vi "20220815-335-write temppoint.vi"() -> ()   [LabVIEW 2019]
doc: "This example VI demonstrates the proper use of the Configure Curve Header and Configure Curve Point VIs. It allows the user to write a curve header, a curve point, of both."
panel:
  out "当前已经写入（点数）":i32
  in  "曲线序号":string="59"
  in  "VISA resource name":refnum<visa-resource-name>
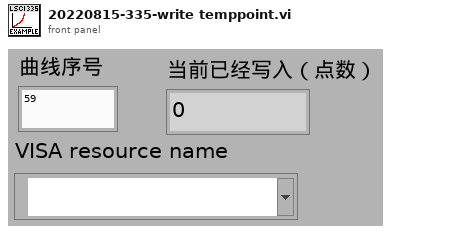
[diagram p1: front panel]
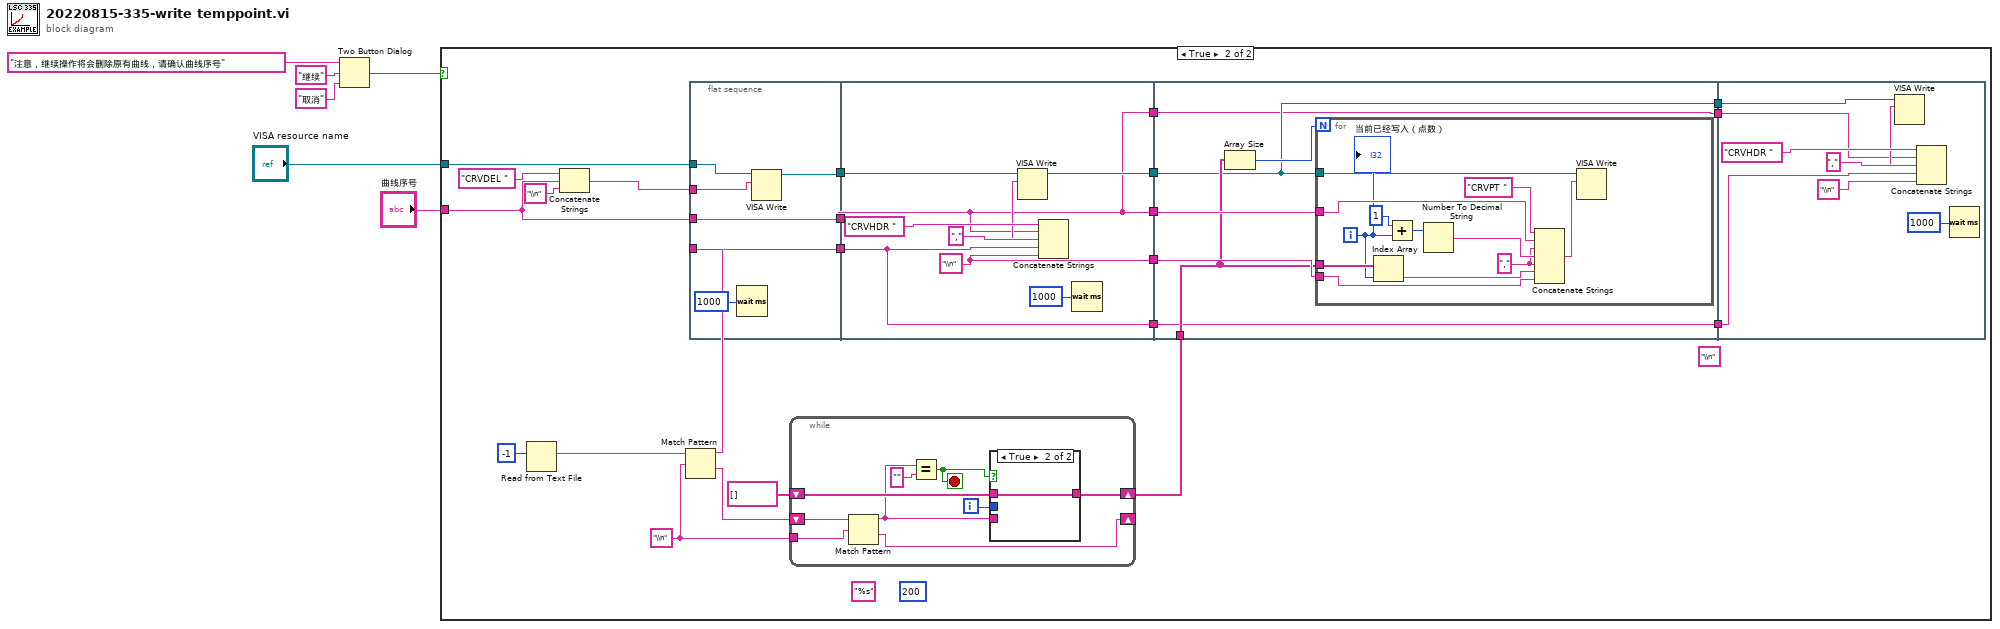
[diagram p0: block diagram]
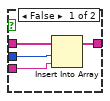
[diagram p3: hidden frame]
diagram:
  n1 = Two Button Dialog(message="注意，继续操作将会删除原有曲线，请确认曲线序号", 1:"取消" ("F button name (\"Cancel\")"), 2:"继续" ("T button name (\"OK\")")) -> (T button?=w6:bool)
  n2 = case shown="True" w6 {
    tunnel: "曲线序号" -> [_ w22]
    tunnel: "VISA resource name" -> [_ w12]
    frame False {
    }
    frame True {
      (unwired) 200
      (unwired) "%s" ("format string")
      (unwired) "\\n" ("delimiter (Tab)")
      w20 = "\\n" ("regular expression")
      n3 = Read from Text File(count=-1) -> (text=w28:string)  [unwired: 3 in, 3 out]
      n4 = Concatenate Strings("CRVDEL " ("string"), w22, "\\n" ("string")) -> (w13:string)
      n5 = Match Pattern(string=w28, regular expression=w20) -> (before substring=w27:string, after substring=w21:string)  [unwired: 1 in, 2 out]
      n6 = flat-sequence {
        tunnel: w22 -> [w48]
        tunnel: w27 -> [w49]
        tunnel: [w49] -> w16
        tunnel: [w48] -> w15
        tunnel: [w45] -> w14
        tunnel: w13 -> [w47]
        tunnel: w12 -> [w46]
        tunnel: [w51] -> w26
        tunnel: [w56] -> w25
        tunnel: [w53] -> w17
        tunnel: w16 -> [w50]
        tunnel: w15 -> [w51]
        tunnel: w14 -> [w55]
        tunnel: [w51] -> w10
        tunnel: [w50] -> w7
        tunnel: w26 -> [w65]
        tunnel: w25 -> [w64]
        tunnel: w18 -> [w63]
        tunnel: w17 -> [w61]
        tunnel: [w61] -> w11
        tunnel: w10 -> [w60]
        tunnel: [w60] -> w9
        tunnel: [w59] -> w8
        tunnel: w7 -> [w59]
        tunnel: w11 -> [w80]
        tunnel: w9 -> [w79]
        tunnel: w8 -> [w78]
        frame #0 {
          n7 = Wait (ms)(milliseconds to wait=u32 1000) -> ()  [unwired: 1 out]
          n8 = VISA Write(VISA resource name=w46, write buffer=w47) -> (VISA resource name out=w45:refnum<visa-resource-name>)  [unwired: 1 in, 2 out]
        }
        frame #1 {
          w56 = "\\n" ("string")
          n9 = Concatenate Strings("CRVHDR " ("write buffer"), w51, "," ("string"), w50, w56) -> (w54:string)
          n10 = VISA Write(VISA resource name=w55, write buffer=w54) -> (VISA resource name out=w53:refnum<visa-resource-name>)  [unwired: 1 in, 2 out]
          n11 = Wait (ms)(milliseconds to wait=u32 1000) -> ()  [unwired: 1 out]
        }
        frame #2 {
          n12 = Array Size(array=w63) -> (size(s)=w62:i32)
          n13 = for {
            N: w62 -> [_]
            tunnel: w63 -> [w77]
            tunnel: w65 -> [w72]
            tunnel: w64 -> [w68]
            tunnel: w61 -> [w67]
            i -> [w70]
            w71 = "," ("string")
            n14 = Index Array(array=w77, index=w70) -> (element=w69:string)
            n15 = Add(x=1, y=w70) -> (x+y=w74:i32)
            n16 = Number To Decimal String(number=w74) -> (decimal integer string=w73:string)  [unwired: 1 in]
            n17 = Concatenate Strings("CRVPT " ("string"), w72, w71, w73, w71, w69, w68) -> (w66:string)
            n18 = VISA Write(VISA resource name=w67, write buffer=w66) -> ()  [unwired: 1 in, 3 out]
            "当前已经写入（点数）" <- w70
          }
        }
        frame #3 {
          n19 = Concatenate Strings("CRVHDR " ("write buffer"), w79, "," ("string"), w78, "\\n" ("string")) -> (w82:string)
          n20 = VISA Write(VISA resource name=w80, write buffer=w82) -> ()  [unwired: 1 in, 3 out]
          n21 = Wait (ms)(milliseconds to wait=u32 1000) -> ()  [unwired: 1 out]
        }
      }
      n22 = while {
        shift-right: [w36] -> _
        shift-left: w21 -> [w38]
        tunnel: w20 -> [w37]
        shift-right: [w33] -> w18
        shift-left: string[] [] ("after substring 2") -> [w35]
        i -> [w34]
        stop <- w30 stop-if-true
        n23 = Match Pattern(string=w38, regular expression=w37) -> (before substring=w32:string, after substring=w36:string)  [unwired: 1 in, 2 out]
        n24 = Equal?(x=w32, y="") -> (x = y?=w30:bool)
        n25 = case shown="True" w30 {
          tunnel: w35 -> [w42 w43]
          tunnel: w34 -> [w41 _]
          tunnel: [w40 w43] -> w33
          tunnel: w32 -> [w39 _]
          frame False {
            n26 = Insert Into Array(array=w42, index=w41, new element=w39) -> (w40:string[])
          }
          frame True {
          }
        }
      }
    }
  }
